vi "main.vi"() -> ()   [LabVIEW 2020]
uses:
  <vilib>/sklein/WebView2/Webview2 Control/WebView2 Control.xctl
  <vilib>/sklein/WebView2/Webview2 Control/Paths.ctl
  <vilib>/MediaMongrels Ltd/WebSockets/Sockets/VISA TCP Listener/VISA TCP Listener.lvclass
  <vilib>/MediaMongrels Ltd/WebSockets/WebSockets/WebSocket Server/WebSocket Server.lvclass
panel:
  in  "WebView2 Control":string(xcontrol)
  out "Received Data":string
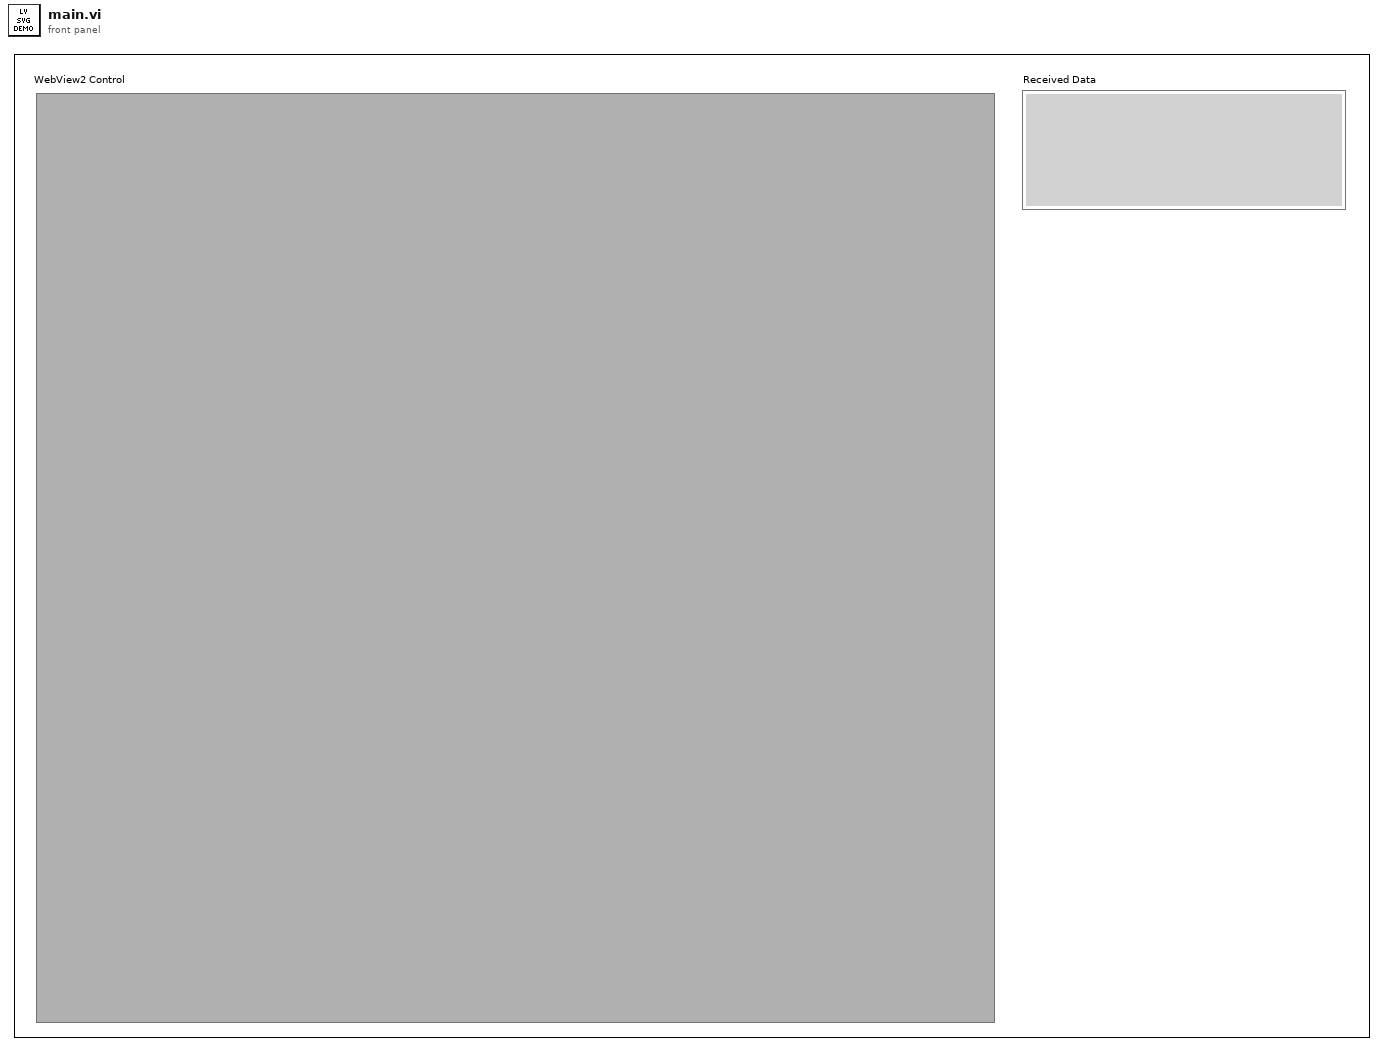
[diagram p1: front panel]
types:
  T1 = typedef "WebView2 Control.xctl/Paths.ctl" = cluster{"Webview2 Native":path, "Edge Application":path, "User Data":path}
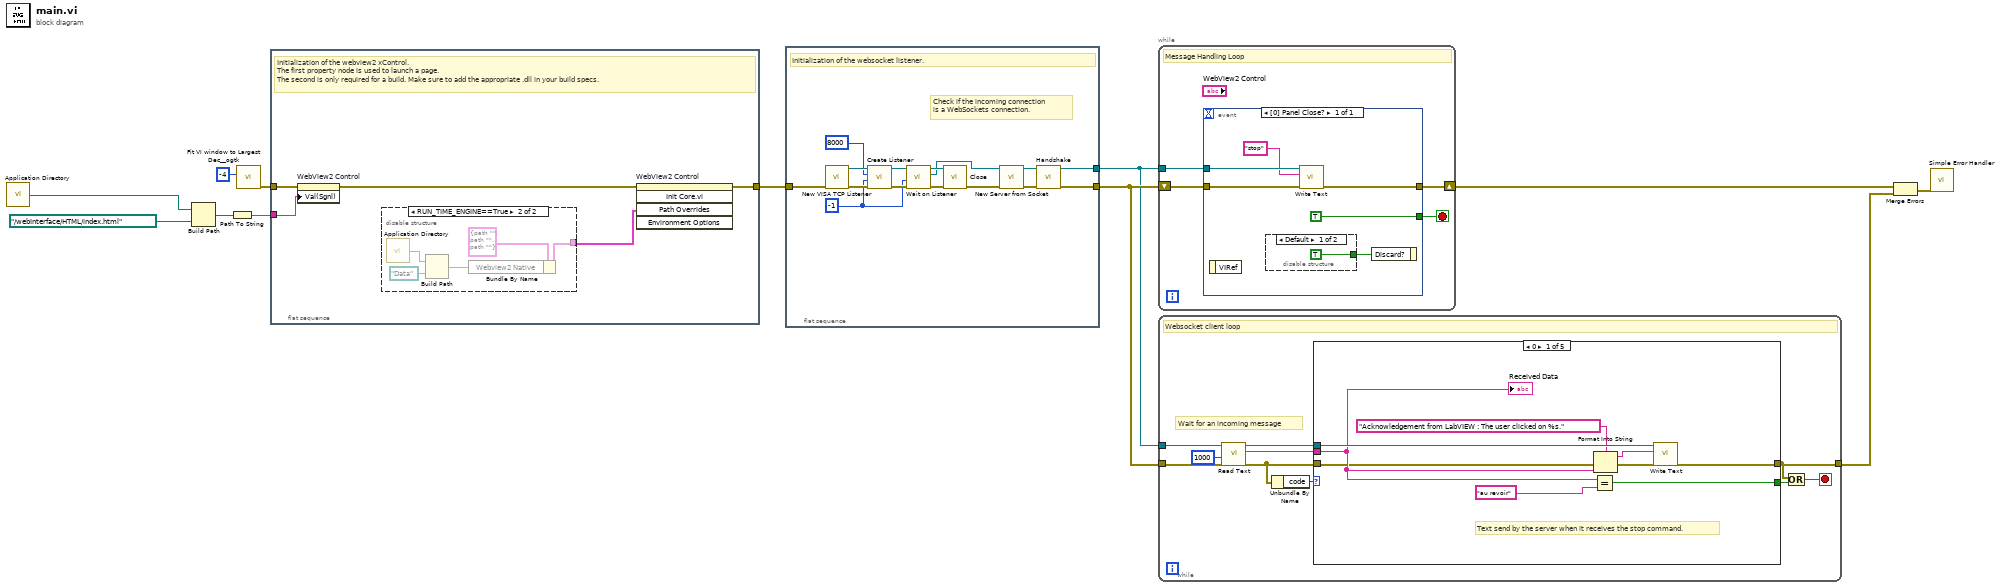
[diagram p0: block diagram]
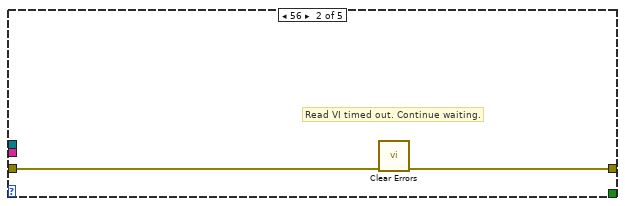
[diagram p3: hidden frame]
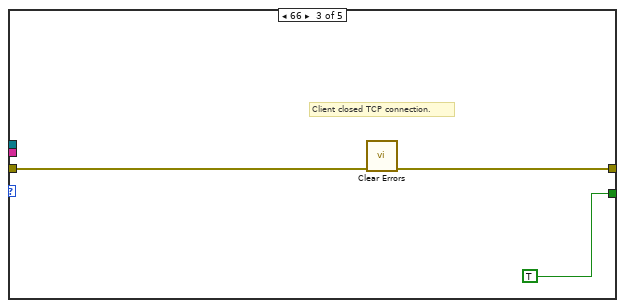
[diagram p4: hidden frame]
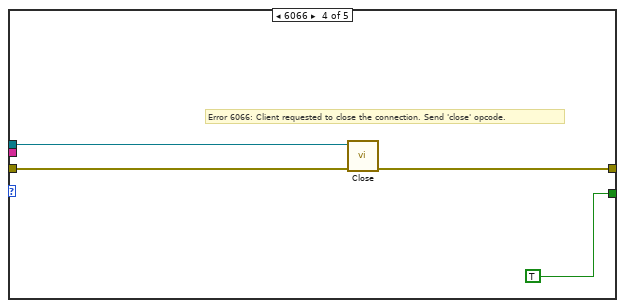
[diagram p5: hidden frame]
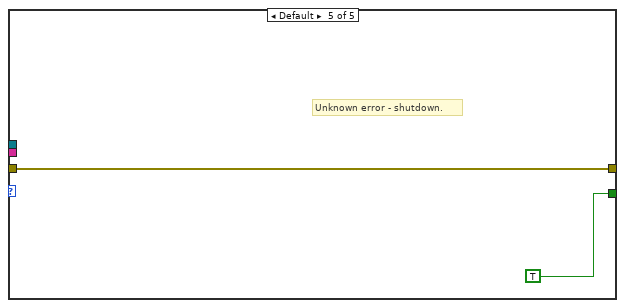
[diagram p6: hidden frame]
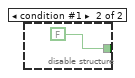
[diagram p7: hidden frame]
diagram:
  n1 = call <vilib>:"Application Directory.vi"() -> ("Application Directory"=w12:path)
  n2 = Build Path(base path=w12, name or relative path=path "../webInterface/HTML/index.html") -> (appended path=w11:path)
  n3 = Path To String(path=w11) -> (string=w6:string)
  n4 = call <userlib>:"Fit VI window to Largest Dec__ogtk.vi"("border spacing (2 px)"=-4) -> ("error out"=w2:errorcluster)  [unwired: 5 in, 1 out]
  n5 = flat-sequence {
    tunnel: w6 -> [w17]
    tunnel: [w15] -> w3
    tunnel: w2 -> [w13]
    frame #0 {
      # "Initialization of the webview2 xControl.\nThe first property node is used to launch a page.\nThe second is only required for a build. Make sure to add the appropriate .dll in your build specs."
      n6 = property on="WebView2 Control" class="WebView2 Control (strict)"(error in=w13, "Val(Sgnl)"=w17) -> (error out=w16:errorcluster)  [unwired: 1 in, 1 out]
      n7 = disable-structure shown="RUN_TIME_ENGINE==True" {
        disable-tunnel: [_ w21] -> w14
        frame condition #0 (active) {
        }
        frame condition #1 {
          n8 = call <vilib>:"Application Directory.vi"() -> ("Application Directory"=w20:path)
          n9 = Build Path(base path=w20, name or relative path=path "Data") -> (appended path=w18:path)
          n10 = Bundle By Name(cluster=T1 {"Webview2 Native"=path "", "Edge Application"=path "", "User Data"=path ""} ("Path Overrides"), "Webview2 Native"=w18) -> (w21:T1)
        }
      }
      n11 = invoke on="WebView2 Control" class="WebView2 Control (strict)" method="Init Core.vi"(error in=w16, "Path Overrides"=w14) -> (error out=w15:errorcluster)  [unwired: 3 in, 4 out]
    }
  }
  n12 = flat-sequence {
    tunnel: [w25] -> w9
    tunnel: [w24] -> w5
    tunnel: w3 -> [w23]
    frame #0 {
      w28 = -1 ("timeout ms (25000)")
      # "Check if the incoming connection\nis a WebSockets connection."
      # "Initialization of the websocket listener."
      n13 = call <vilib>:"New VISA TCP Listener.vi"("error in (no error)"=w23) -> ("error out"=w34:errorcluster, "VISA TCP Listener out"=w35:refnum<class "VISA TCP Listener.lvclass">)  [unwired: 9 in]
      n14 = call-dynamic "Create Listener.vi"("error in (no error)"=w34, "timeout ms (5000)"=w28, "Port"=u16 8000 ("port"), "VISA TCP Listener in"=w35) -> ("error out"=w32:errorcluster, "VISA TCP Listener out"=w30:refnum<class "VISA TCP Listener.lvclass">)  [unwired: 6 in]
      n15 = call-dynamic "Wait on Listener.vi"("error in (no error)"=w32, "timeout ms (5000)"=w28, "VISA TCP Listener in"=w30) -> ("error out"=w33:errorcluster, "Socket out"=w27:refnum<class "Socket.lvclass">, "VISA TCP Listener out"=w31:refnum<class "VISA TCP Listener.lvclass">)  [unwired: 6 in]
      n16 = call-dynamic "Close.vi"("error in (no error)"=w33, "VISA TCP Listener in"=w31) -> ("error out"=w26:errorcluster)  [unwired: 9 in]
      n17 = call <vilib>:"New Server from Socket.vi"("error in (no error)"=w26, "Socket"=w27) -> ("error out"=w36:errorcluster, "WebSocket Server out"=w37:refnum<class "WebSocket Server.lvclass">)  [unwired: 8 in]
      n18 = call-dynamic "Handshake.vi"("error in (no error)"=w36, "WebSocket Connection in"=w37) -> ("error out"=w25:errorcluster, "WebSocket Connection out"=w24:refnum<class "WebSocket Server.lvclass">)  [unwired: 8 in]
    }
  }
  n19 = while {
    shift-right: [w39] -> w8
    shift-left: w9 -> [w40]
    tunnel: w5 -> [w38]
    stop <- w41 stop-if-true
    # "Message Handling Loop"
    n20 = event shown="[0] Panel Close?" {
      selector: _ -> [_]
      dyn-events: _ -> [_]
      timeout: _ -> [_]
      tunnel: [TRUE] -> w41
      tunnel: w40 -> [w44]
      tunnel: [w43] -> w39
      tunnel: w38 -> [w45]
      event Panel Close? {
        n21 = event-data() -> ()  [unwired: 1 in, 1 out]
        n22 = disable-structure shown="Default" {
          disable-tunnel: [TRUE FALSE] -> w47
          frame condition #0 (active) {
          }
          frame condition #1 {
          }
        }
        n23 = call-dynamic "Write Text.vi"("error in (no error)"=w44, "String Data"="stop", "WebSocket in"=w45) -> ("error out"=w43:errorcluster)  [unwired: 7 in, 1 out]
        n24 = event-data("Discard?"=w47) -> ()  [unwired: 1 in, 1 out]
      }
    }
  }
  n25 = while "Read Loop" {
    tunnel: w5 -> [w59]
    tunnel: [w52] -> w10
    tunnel: w9 -> [w53]
    stop <- w50 stop-if-true
    # "Wait for an incoming message"
    # "Websocket client loop"
    n26 = call-dynamic "Read Text.vi"("error in (no error)"=w53, "timeout ms (5000)"=1000 ("timeout ms (25000)"), "WebSocket in"=w59) -> ("error out"=w54:errorcluster, "Data"=w56:string, "WebSocket out"=w55:refnum<class "WebSocket Server.lvclass">)  [unwired: 6 in]
    n27 = Unbundle By Name(w54) -> ("code"=w57:i32)
    n28 = case shown="0" w57 {
      tunnel: w56 -> [w64 _ _ _ _]
      tunnel: [w65 _ TRUE TRUE TRUE] -> w51
      tunnel: w55 -> [w68 _ _ w77 _]
      tunnel: w54 -> [w62 w70 w72 w75 w78]
      tunnel: [w67 w69 w71 w74 w78] -> w52
      frame 0 {
        # "Text send by the server when it receives the stop command."
        n29 = Equal?(x=w64, y="au revoir") -> (x = y?=w65:bool)
        n30 = Format Into String(format string="Acknowledgement from LabVIEW : The user clicked on %s.", error in=w62, w64) -> (resulting string=w60:string, error out=w61:errorcluster)  [unwired: 1 in]
        n31 = call-dynamic "Write Text.vi"("error in (no error)"=w61, "String Data"=w60, "WebSocket in"=w68) -> ("error out"=w67:errorcluster)  [unwired: 7 in, 1 out]
        "Received Data" <- w64
      }
      frame 56 {
        # "Read VI timed out. Continue waiting."
        n32 = call <vilib>:"Clear Errors.vi"("error in (no error)"=w70) -> ("error out"=w69:errorcluster)  [unwired: 5 in, 1 out]
      }
      frame 66 {
        # "Client closed TCP connection."
        n33 = call <vilib>:"Clear Errors.vi"("error in (no error)"=w72) -> ("error out"=w71:errorcluster)  [unwired: 5 in, 1 out]
      }
      frame 6066 {
        # "Error 6066: Client requested to close the connection. Send 'close' opcode."
        n34 = call-dynamic "Close.vi"("error in (no error)"=w75, "WebSocket in"=w77) -> ("error out"=w74:errorcluster)  [unwired: 9 in]
      }
      frame Default {
        # "Unknown error - shutdown."
      }
    }
    n35 = Or(x=w52, y=w51) -> (x .or. y?=w50:bool)
  }
  n36 = Merge Errors(w8, w10) -> (w4:errorcluster)
  n37 = call <vilib>:"Simple Error Handler.vi"("error in (no error)"=w4) -> ()  [unwired: 4 in, 5 out]
